vi "Power_Query.vi"(8 "error in (no error)":errorcluster, 10 "CMD":string, 11 "connection ID":refnum<k5>) -> (0 "error out":errorcluster, 2 "Read Buffer":string, 3 "connection ID out":refnum<k5>)   [LabVIEW 2020]
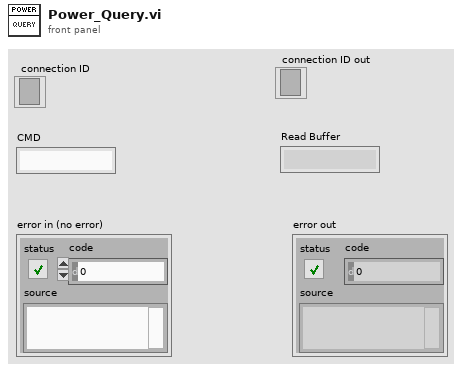
[diagram p1: front panel]
types:
  T1 = enum16{"Standard", "Buffered", "CRLF", "Immediate"}
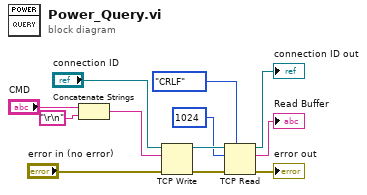
[diagram p0: block diagram]
diagram:
  n1 = Concatenate Strings("CMD", "\r\n") -> (w1:string)
  n2 = TCP Write(connection ID="connection ID", data in=w1, error in (no error)="error in (no error)") -> (connection ID out=w10:refnum<k5>, error out=w11:errorcluster)  [unwired: 1 in, 1 out]
  n3 = TCP Read(connection ID=w10, bytes to read=1024, error in (no error)=w11, 7:T1."CRLF" ("mode (standard)")) -> (connection ID out=→"connection ID out":refnum<k5>, data out=→"Read Buffer":string, error out=→"error out":errorcluster)  [unwired: 1 in]
